vi "Has Parent Ref.vi"(8 "error in (no error)":errorcluster, 11 "Transform Ref in":refnum<vi>) -> (0 "error out":errorcluster, 2 "Has Parent":bool, 3 "Transform Ref out":refnum<vi>)   [LabVIEW 2022 SP3, in "Transform.lvclass"]
uses:
  Transform.lvclass
  Transform.lvclass/Transform.ctl
  D:/Programowanie/Studia/Labview/CollisionSimulator/Project/Engine/Objects/Components/Component/Component.lvclass
  D:/Programowanie/Studia/Labview/CollisionSimulator/Project/Engine/Objects/Components/Transform/Transform.lvclass
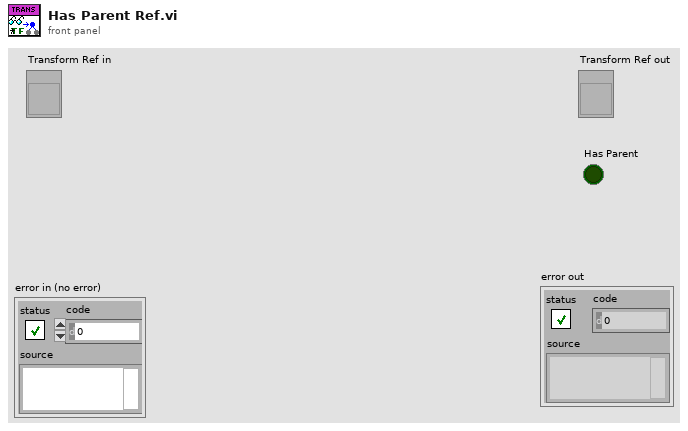
[diagram p1: front panel]
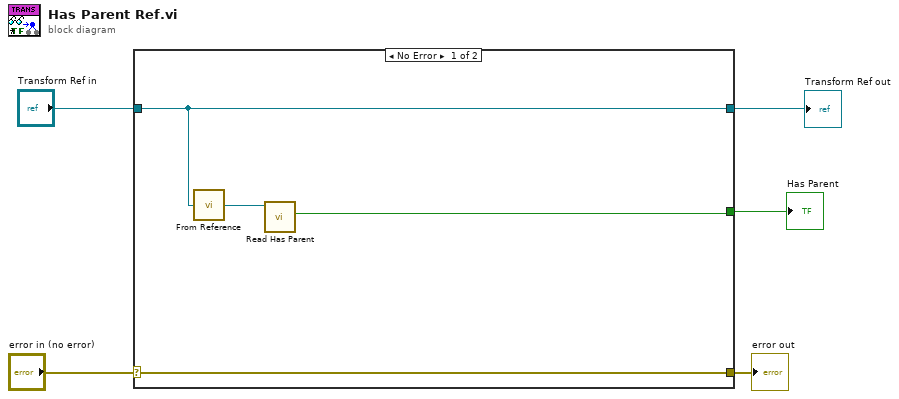
[diagram p0: block diagram]
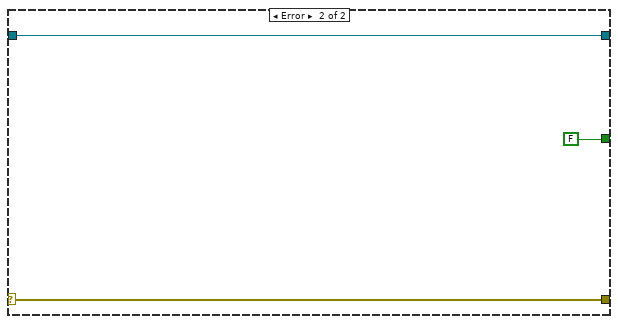
[diagram p2: hidden frame]
diagram:
  n1 = case shown="No Error" "error in (no error)" {
    selector: "error in (no error)" -> [w9 w12]
    tunnel: [w9 w12] -> w4
    tunnel: [w8 w11] -> w2
    tunnel: "Transform Ref in" -> [w8 w11]
    tunnel: [w6 FALSE] -> w1
    frame No Error {
      n2 = call "From Reference.vi"("Transform Ref in"=w8) -> ("Transform out"=w7:refnum<class "Transform.lvclass">)
      n3 = call "Read Has Parent.vi"("Transform in"=w7) -> ("Has Parent"=w6:bool)  [unwired: 8 in, 2 out]
    }
    frame Error {
    }
  }
  "error out" <- w4
  "Transform Ref out" <- w2
  "Has Parent" <- w1
